vi "SPIFreSet.vi"(8 "error in (no error)":errorcluster caption="错误输入（无错误）", 10 "Frequency(Hz)":i32(ring)=9600 items=["110"=110, "150"=150, "300"=300, "600"=600, "1200"=1200, "2400"=2400, "4800"=4800, "9600"=9600, "14400"=14400, "19200"=19200, "28800"=28800, "38400"=38400, "56000"=56000, "57600"=57600, "115200"=115200, "128000"=128000, "153600"=153600, "230400"=230400, "256000"=256000, "406800"=406800, "921600"=921600], 11 "handle":u64) -> (0 "error out":errorcluster caption="错误输出", 2 "function return":i32, 3 "handle out":u64)   [LabVIEW 2018]
doc: "Set pos. or neg. Supply voltage"
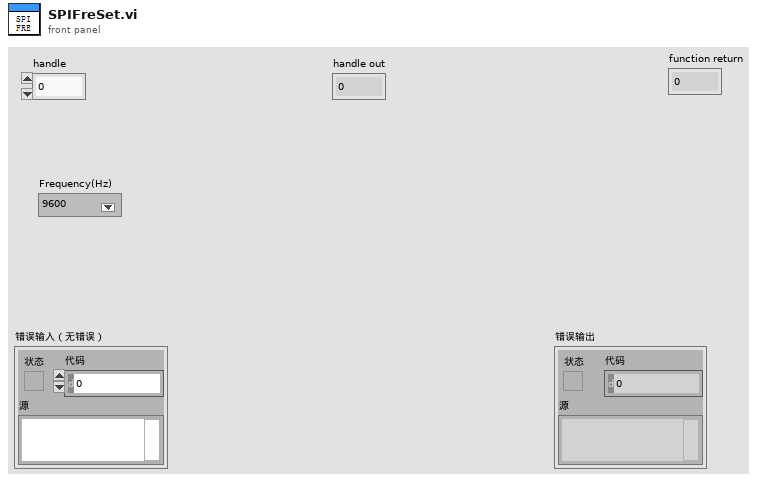
[diagram p1: front panel]
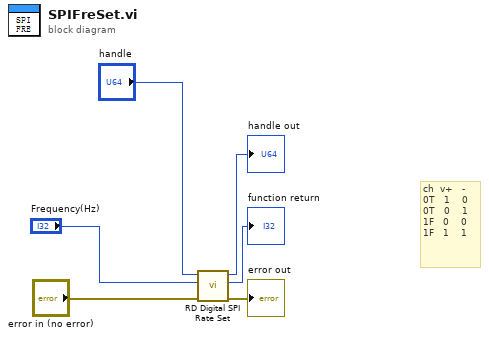
[diagram p0: block diagram]
diagram:
  # "ch  v+   -\n0T   1    0\n0T   0    1\n1F   0    0\n1F   1    1"
  n1 = call "RD Digital SPI Rate Set.vi"("error in (no error)"="error in (no error)", "rate"="Frequency(Hz)", "handle"="handle") -> ("error out"=→"error out":errorcluster, "function return"=→"function return":i32, "handle out"=→"handle out":u64)  [unwired: 6 in]
